vi "Test_Run All Tests.vi"(8 "error in":errorcluster, 9 "Modules":T7, 10 "Part Number":T9, 11 "Test Selection":T8) -> (0 "error out":errorcluster)   [LabVIEW 2025]
uses:
  Classes/Solenoid/Solenoid Selector.ctl
  Controls/Test list.ctl
  Controls/tests tab control.ctl
  Controls/Graphs/XY Graph_Transparent.ctl
  Controls/Test Results/Test Pass Fail.ctl
  Controls/Test Results/Results Table.ctl
  Controls/Numeric Voltage.ctl
  Controls/Numeric Current.ctl
  Classes/Solenoid/Solenoid.lvclass
  Classes/EVI 79/EVI 79.lvclass
  C:/Users/grove/Desktop/LabVIEW/Git/atp-station/Classes/Solenoid/Solenoid.lvclass
  Test_Calculate Wear-in.vi
  Test_Calculate Drop-out.vi
  Test_Calculate CRT.vi
  Test_Calculate Pull-in.vi
  Test_Calculate Hold-in.vi
  Test_Calculate ORT.vi
  Libraries/Power Supply/Power Supply.lvlib
  Libraries/USB IO/USB IO.lvlib
panel:
  out "Voltage Chart":dbl(graph)
  out "Current":T1 format="%5.3f A"
  out "Voltage":T2 format="%5.3f V"
  out "result 3":bool
  out "result 2":bool
  out "result":bool
  in  "Table Control":T3=[["Wear-in", "N/A", "N/A", "", "", "", "", ""], ["Drop-out", "N/A", "N/A", "", "", "", "", ""], ["Closing Response Time", "N/A", "N/A", "", "", "", "", ""], ["Pull-in", "N/A", "N/A", "", "", "", "", ""], ["Hold-in", "N/A", "N/A", "", "", "", "", ""], ["Opening Response Time", "N/A", "N/A", "", "", "", "", ""]]
  out "Errors":errorcluster
  in  "Tab Control":T4
  out "Power Supply Output":bool
  out "Cycles":dbl format="%3.0f of"
  out "Total Cycles":dbl format="%3.0f"
  out "Unit On?":bool
  in  "Abort":bool
  out "Drop-out Voltage":T2 format="%5.3f V"
  out "Drop-out Current":T1 format="%5.3f A"
  out "CRT Graph":T5
  out "Closing Response Time":dbl format="%5.3f ms"
  out "Pass? 2":T6 caption="Test Result"
  out "Pull-in Voltage":T2 format="%5.3f V"
  out "Pull-in Current":T1 format="%5.3f A"
  in  "Abort 2":bool
  out "XY Graph":T5
  out "Pass?":T6 caption="Test Result"
  out "Opening Response Time":dbl format="%5.3f ms"
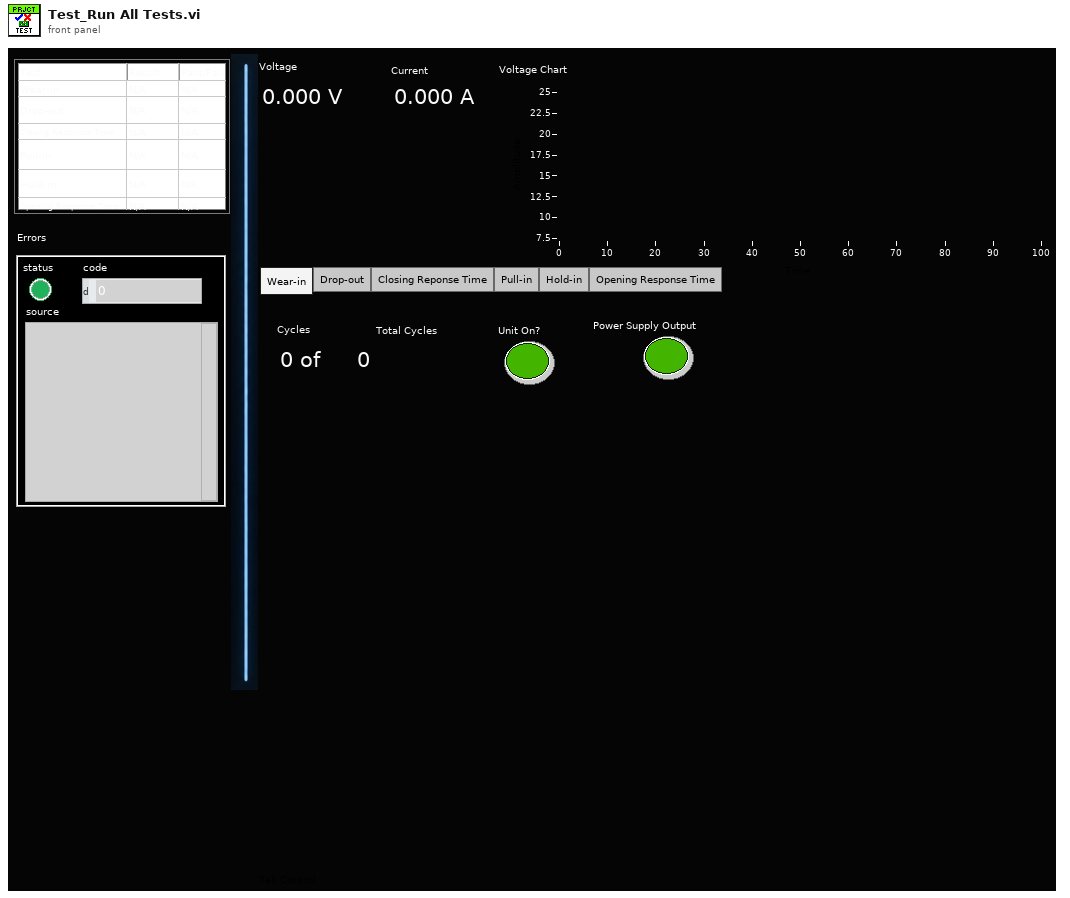
[diagram p1: front panel]
types:
  T1 = typedef "Numeric Current.ctl" = dbl
  T2 = typedef "Numeric Voltage.ctl" = dbl
  T3 = typedef "Results Table.ctl" = string[][]
  T4 = typedef "tests tab control.ctl" = enum32{"Wear-in", "Drop-out", "Closing Reponse Time", "Pull-in", "Hold-in", "Opening Response Time"}
  T5 = typedef "XY Graph_Transparent.ctl" = cluster{dbl[], dbl[]}[]
  T6 = typedef "Test Pass Fail.ctl" = bool
  T7 = cluster{"Module IDs":i32[], "Module Names":string[]}
  T8 = typedef "Test list.ctl" = cluster{"Wear-in":bool, "Drop-out":bool, "Closing Response Time":bool, "Pull-in":bool, "Hold-in":bool, "Opening Response Time":bool}
  T9 = typedef "Solenoid Selector.ctl" = enum16{"Generic Solenoid", "EVI-79"}
  T10 = cluster{"V":dbl, "I":dbl, "Cycles":dbl, "On_Time_ms":dbl, "Off_Time_ms":dbl}
  T11 = cluster{"V":dbl, "I":dbl, "V_reduced":dbl, "V_perturb":dbl, "Plunger_Threshold":dbl, "Plunger_Threshold 2":dbl}
  T12 = cluster{"V":dbl, "I":dbl, "V_increased":dbl, "V_perturb":dbl, "Plunger_Threshold":dbl, "V_MAX":dbl}
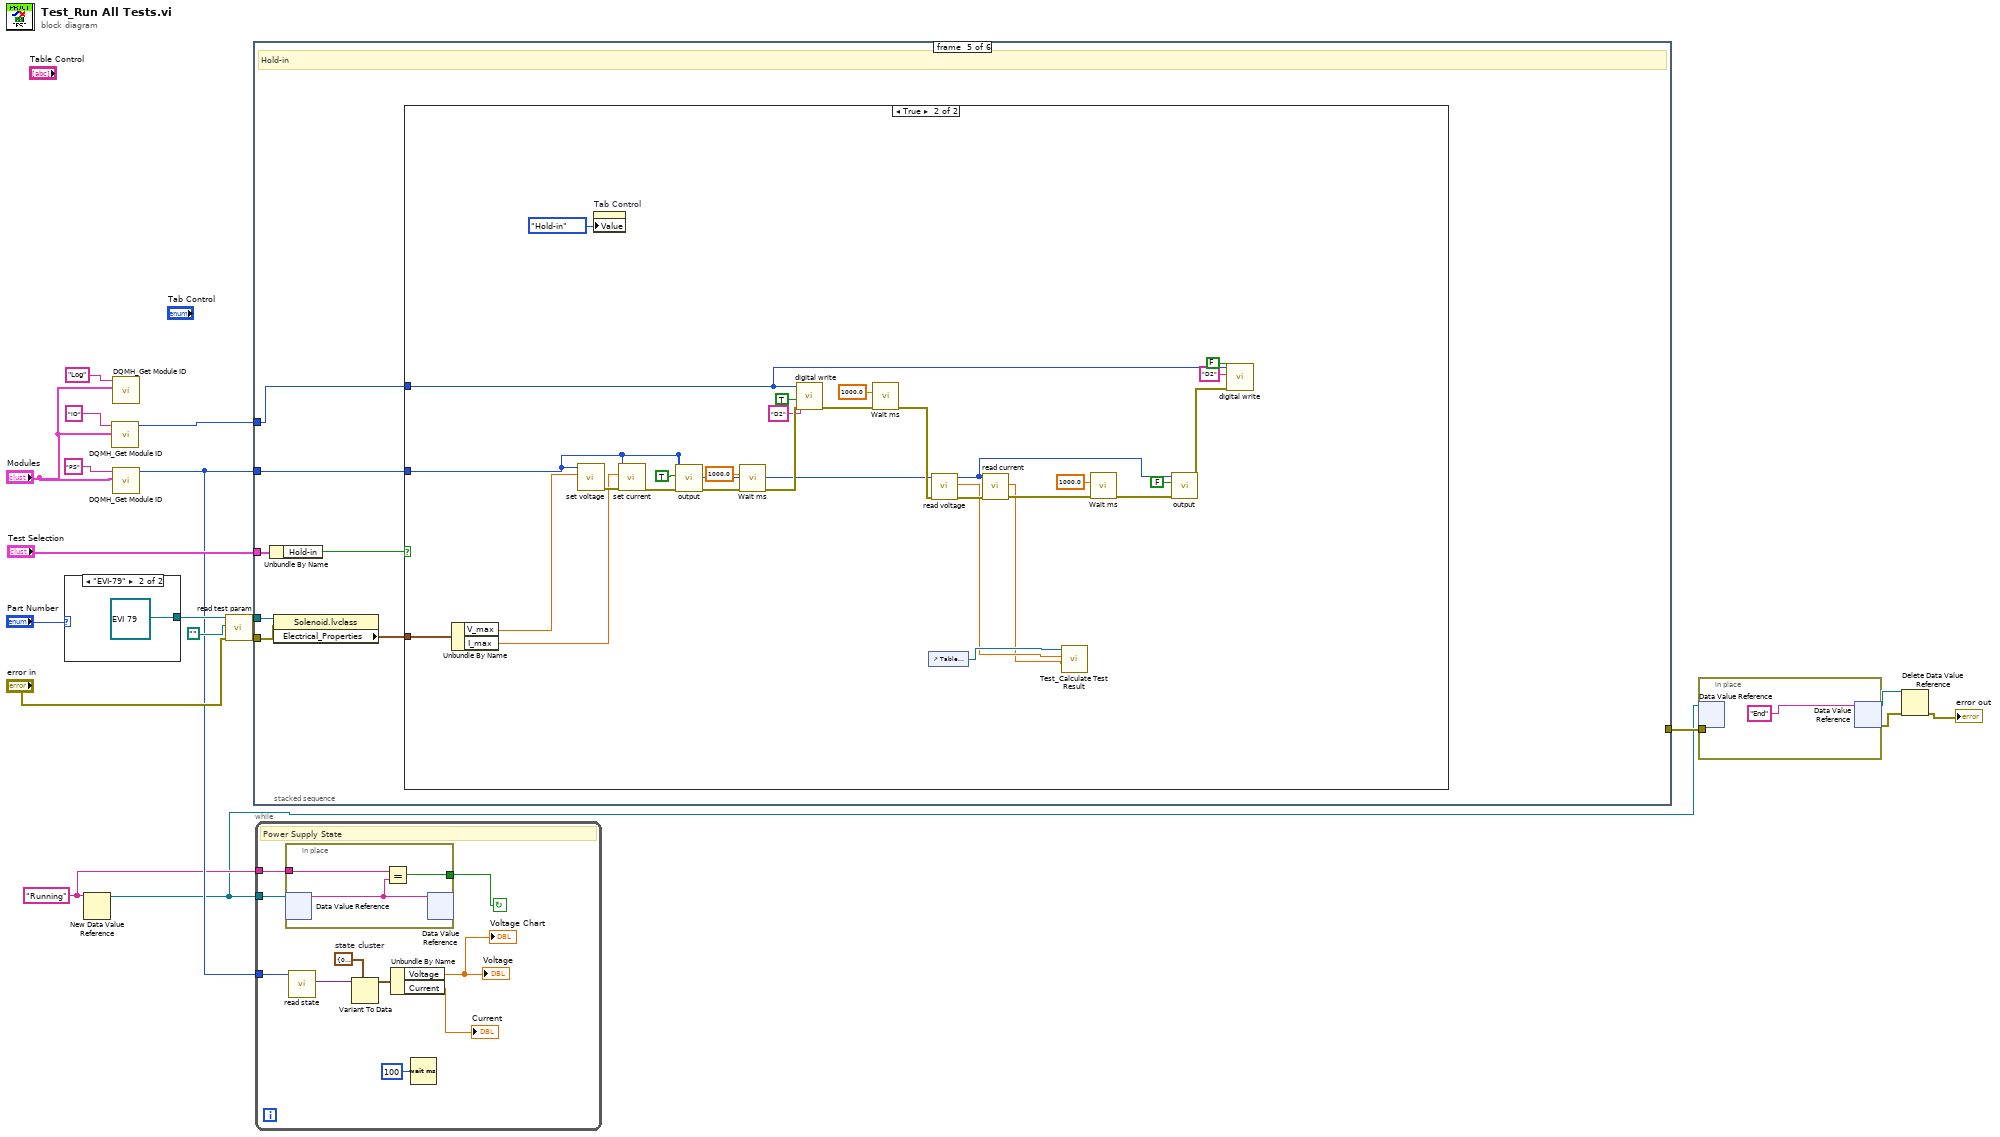
[diagram p0: block diagram]
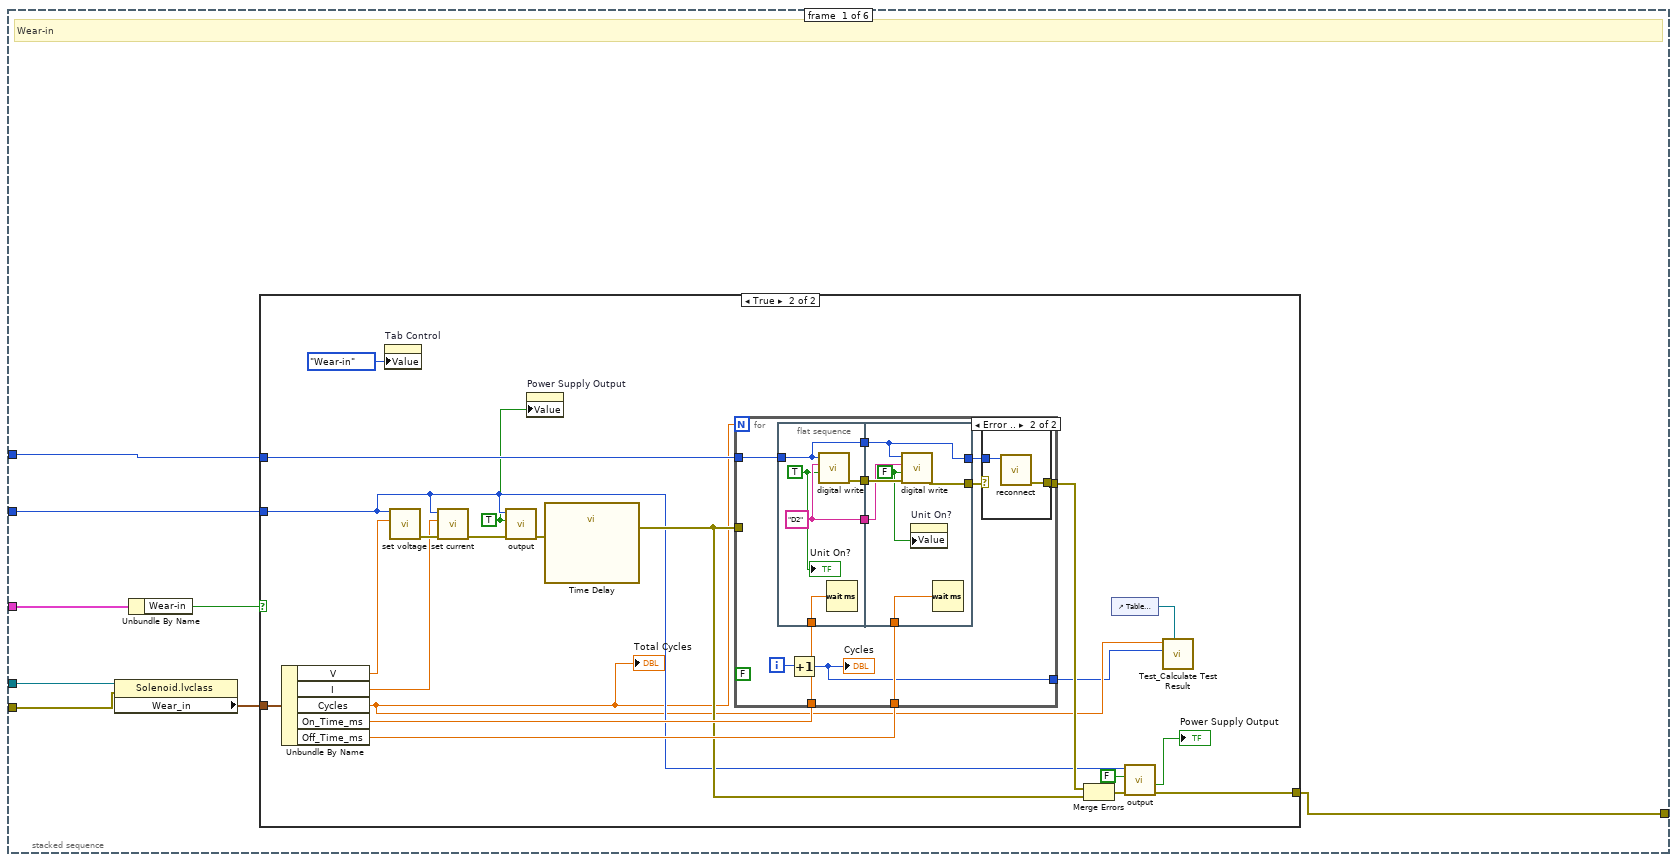
[diagram p2: hidden frame]
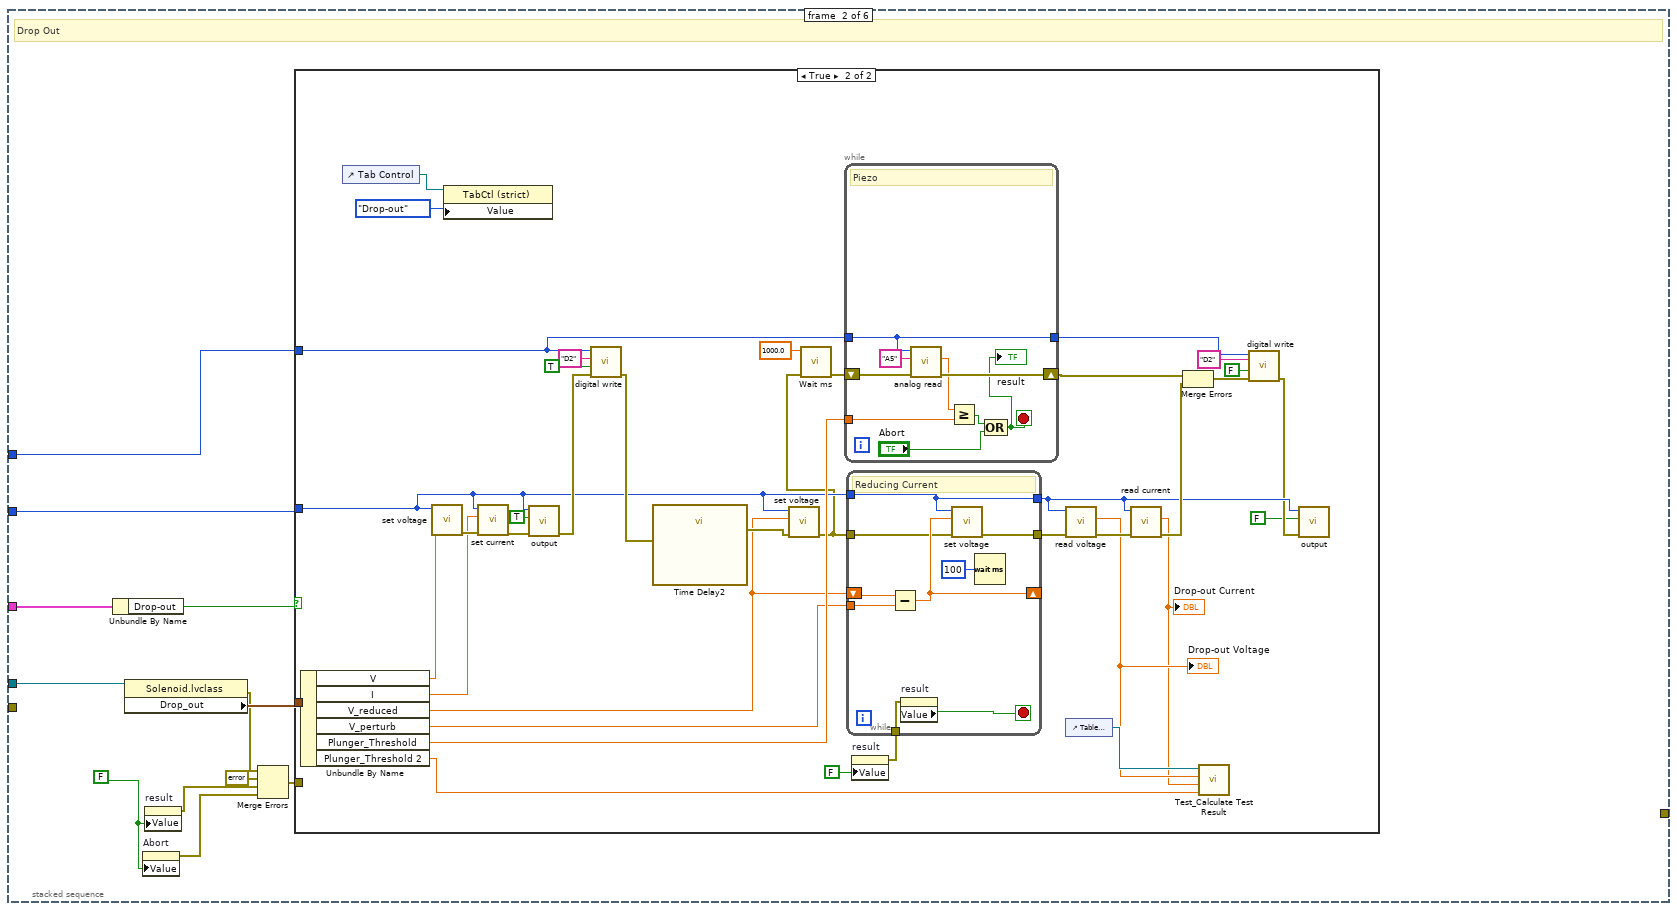
[diagram p5: hidden frame]
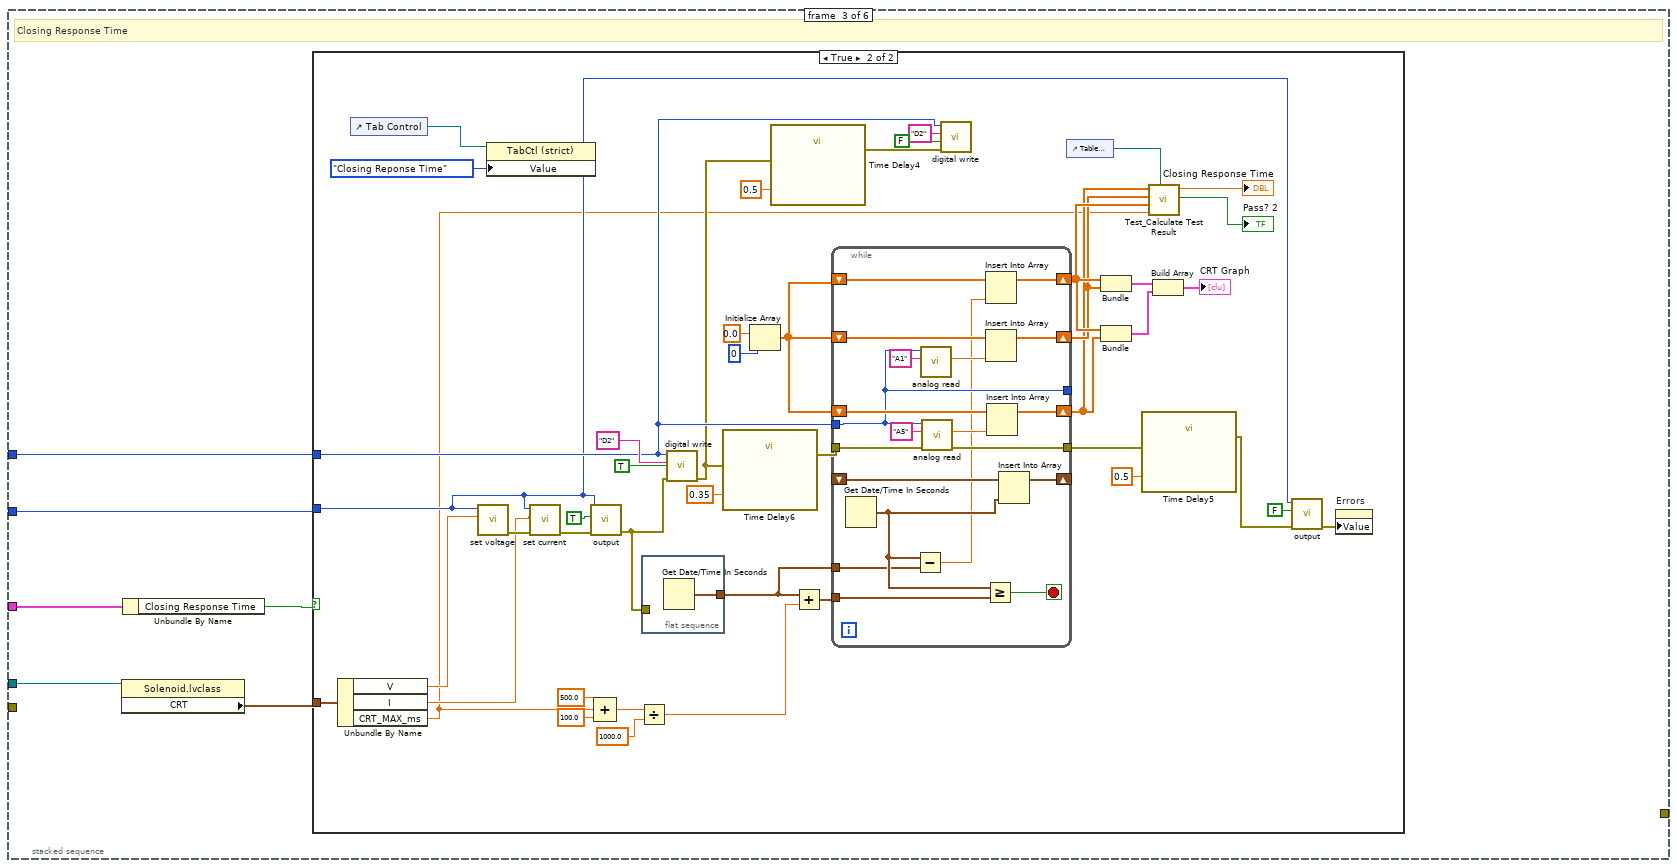
[diagram p7: hidden frame]
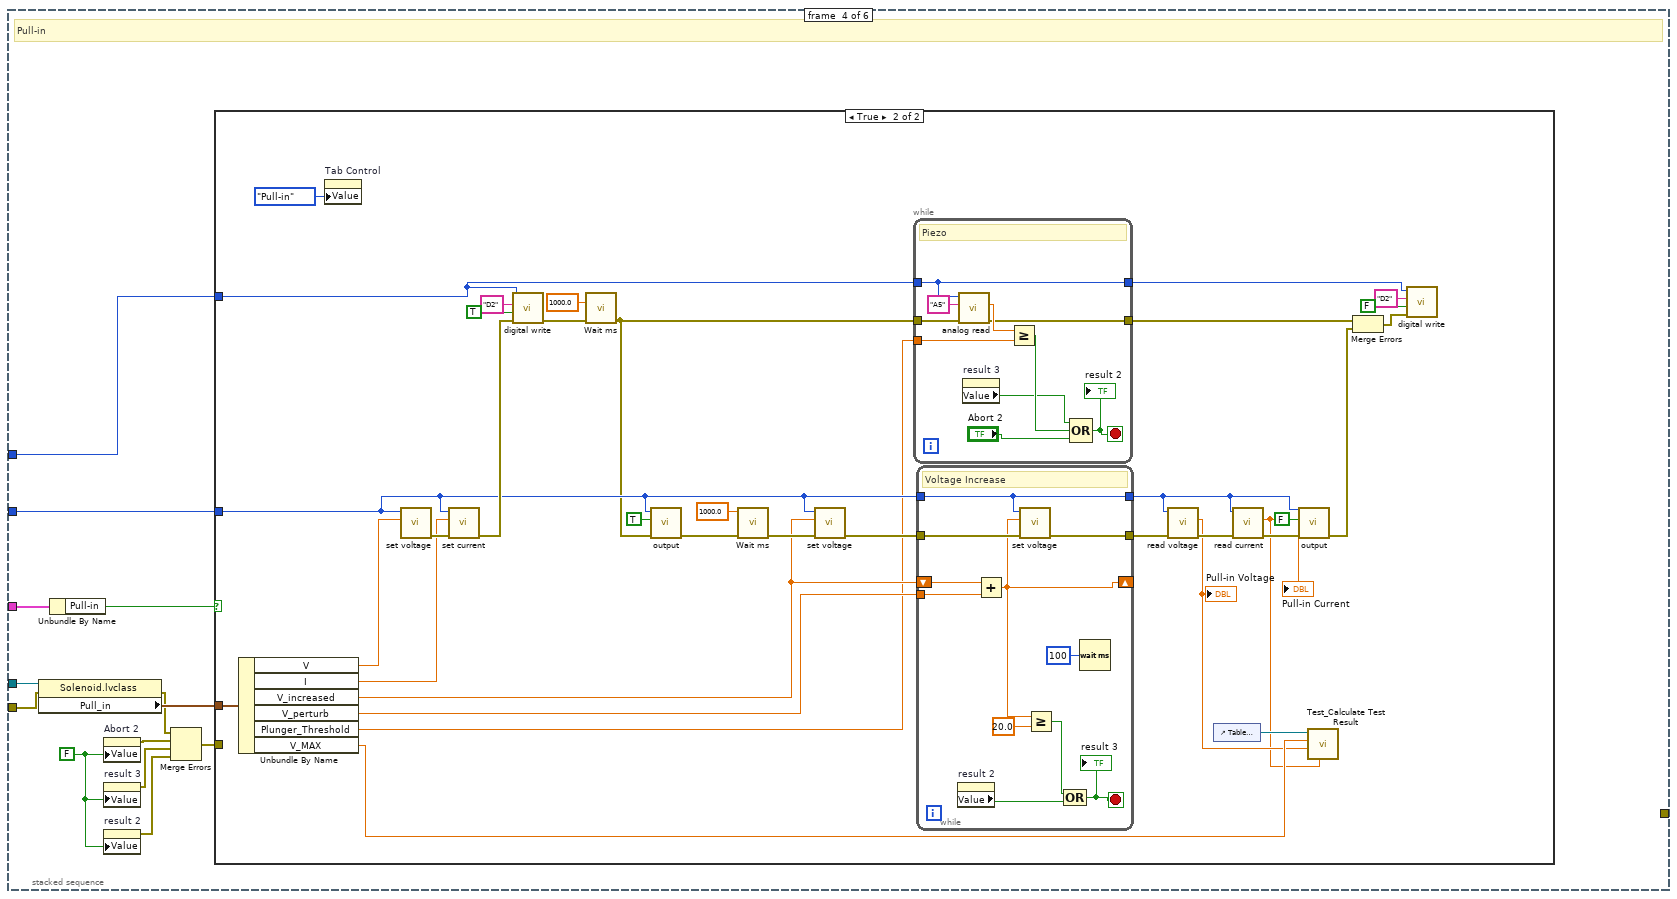
[diagram p9: hidden frame]
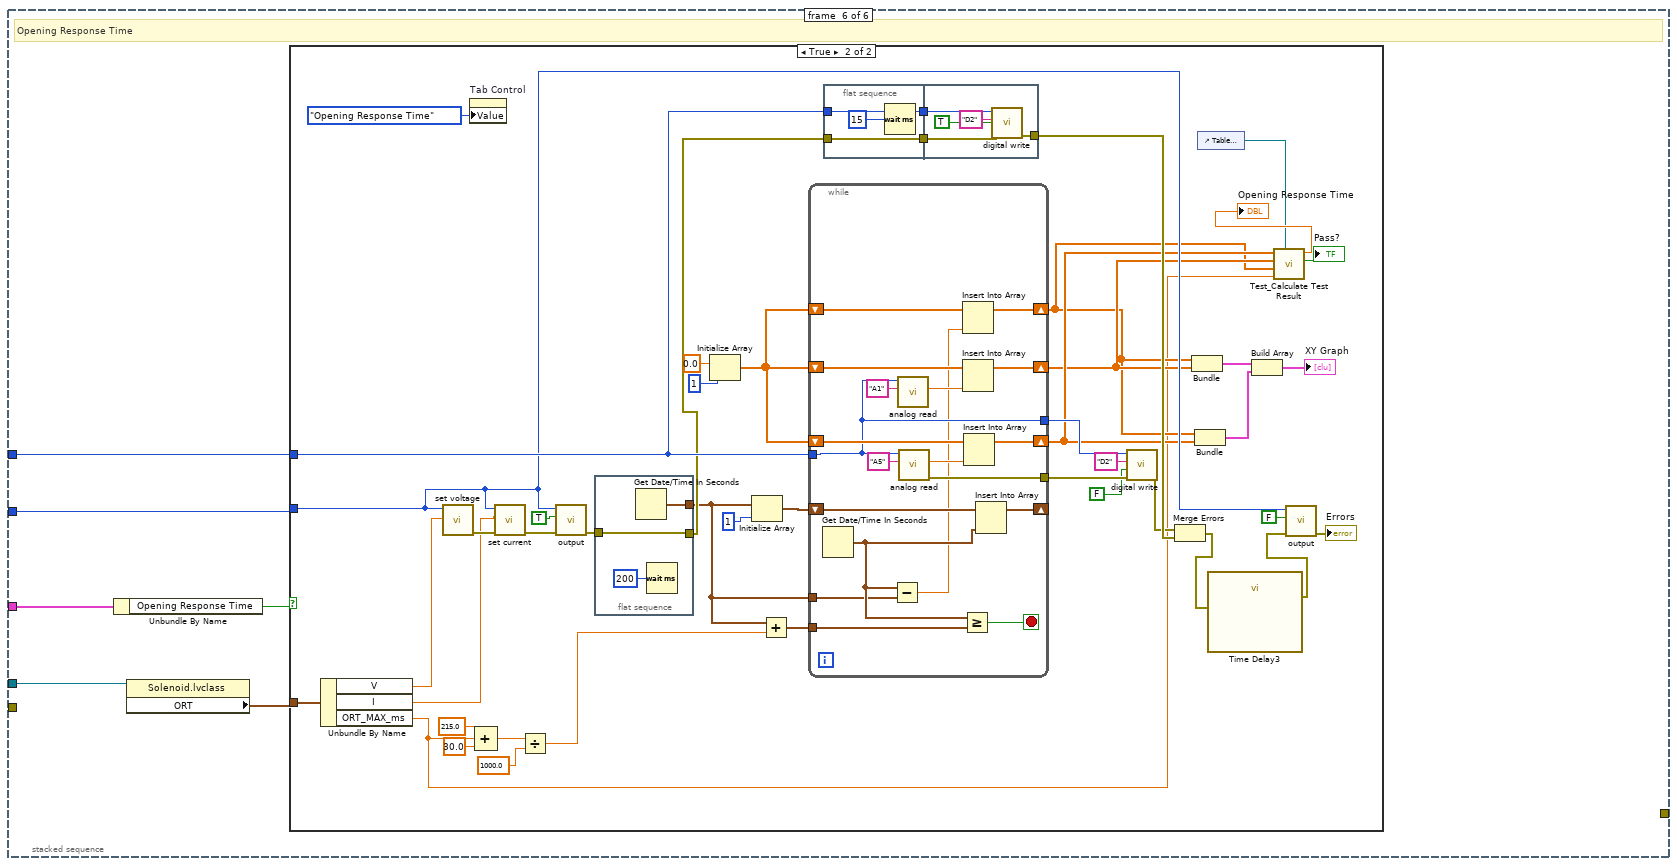
[diagram p12: hidden frame]
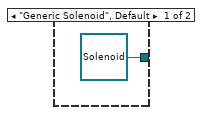
[diagram p14: hidden frame]
diagram:
  w6 = "Running"
  n1 = case shown="\"EVI-79\"" "Part Number" {
    tunnel: [refnum<class "Solenoid.lvclass"> refnum ("Solenoid.lvclass") refnum<class "EVI 79.lvclass"> refnum ("EVI 79.lvclass")] -> w18
    frame "Generic Solenoid", Default {
    }
    frame "EVI-79" {
    }
  }
  n2 = New Data Value Reference(data value=w6) -> (data value reference=w4:refnum<data-value>)  [unwired: 1 in, 1 out]
  n3 = call "DQMH_Get Module ID.vi"("Modules"="Modules", "Module Name"="IO") -> ("Module ID out"=w8:i32)  [unwired: 9 in]
  n4 = call "DQMH_Get Module ID.vi"("Modules"="Modules", "Module Name"="Log") -> ()  [unwired: 9 in, 1 out]
  n5 = call "DQMH_Get Module ID.vi"("Modules"="Modules", "Module Name"="PS") -> ("Module ID out"=w7:i32)  [unwired: 9 in]
  n6 = call-dynamic "read test param.vi"("error in (no error)"="error in", "File Path"=path "", "Solenoid in"=w18) -> ("error out"=w13:errorcluster, "Solenoid out"=w15:refnum<class "Solenoid.lvclass">)  [unwired: 7 in]
  n7 = stacked-sequence {
    tunnel: w15 -> [w27 w85 w147 w226 w290 w326]
    tunnel: "Test Selection" -> [w29 w87 w149 w228 w292 w325]
    tunnel: w13 -> [w26 _ _ w225 w289 _]
    tunnel: w7 -> [w24 w83 w145 w223 w287 w322]
    tunnel: w8 -> [w23 w82 w144 w222 w286 w321]
    tunnel: [w22 _ _ _ _ _] -> w5
    frame #0 {
      # "Wear-in"
      n8 = property class="Solenoid.lvclass"(reference=w27, error in=w26) -> ("Wear_in"=w25:T10)  [unwired: 2 out]
      n9 = Unbundle By Name(w29) -> ("Wear-in"=w28:bool)
      n10 = case shown="True" w28 {
        tunnel: w25 -> [_ w50]
        tunnel: w24 -> [_ w39]
        tunnel: w23 -> [_ w46]
        tunnel: [_ w40] -> w22
        frame False {
        }
        frame True {
          w37 = TRUE ("Output On/Off")
          n11 = Unbundle By Name(w50) -> ("V"=w32:dbl, "I"=w31:dbl, "Cycles"=w35:dbl, "On_Time_ms"=w48:dbl, "Off_Time_ms"=w47:dbl)
          "Total Cycles" <- w35
          n12 = property on="Tab Control" class="TabCtl (strict)"("Value"=tests_tab_control."Wear-in" ("Tab Control")) -> ()  [unwired: 2 in, 2 out]
          n13 = call "set voltage.vi"("Output Voltage"=w32, "Module ID"=w39) -> ("error out"=w49:errorcluster)  [unwired: 8 in, 1 out]
          n14 = call "set current.vi"("error in"=w49, "Output Current"=w31, "Module ID"=w39) -> ("error out"=w45:errorcluster)  [unwired: 7 in, 1 out]
          n15 = call "output.vi"("error in"=w45, "Output On/Off"=w37, "Module ID"=w39) -> ("error out"=w44:errorcluster)  [unwired: 7 in, 1 out]
          n16 = property on="Power Supply Output" class="Bool (strict)"("Value"=w37) -> ()  [unwired: 2 in, 2 out]
          n17 = call "Time Delay"("error in (no error)"=w44) -> ("error out"=w42:errorcluster)  [unwired: 10 in]
          n18 = for {
            N: w35 -> [_]
            tunnel: w48 -> [w61]
            tunnel: w47 -> [w60]
            tunnel: w46 -> [w59]
            tunnel: w42 -> [_]
            tunnel: [w53] -> w43
            tunnel: [w51] -> w34
            i -> [w55]
            (unwired) FALSE ("Power Supply Output")
            n19 = flat-sequence {
              tunnel: w61 -> [w69]
              tunnel: w59 -> [w67]
              tunnel: [w68] -> w58
              tunnel: [w67] -> w57
              tunnel: [w66] -> w56
              tunnel: w60 -> [w73]
              tunnel: w58 -> [w75]
              tunnel: w57 -> [w70]
              tunnel: w56 -> [w74]
              tunnel: [w72] -> w54
              tunnel: [w70] -> w52
              frame #0 {
                w65 = TRUE ("On/Off")
                w66 = "D2" ("Line")
                n20 = call "digital write.vi"("On/Off"=w65, "Line"=w66, "Module ID"=w67) -> ("error out"=w68:errorcluster)  [unwired: 7 in, 1 out]
                n21 = Wait (ms)(milliseconds to wait=w69) -> ()  [unwired: 1 out]
                "Unit On?" <- w65
              }
              frame #1 {
                w71 = FALSE ("On/Off")
                n22 = call "digital write.vi"("error in"=w75, "On/Off"=w71, "Line"=w74, "Module ID"=w70) -> ("error out"=w72:errorcluster)  [unwired: 6 in, 1 out]
                n23 = property on="Unit On?" class="Bool (strict)"("Value"=w71) -> ()  [unwired: 2 in, 2 out]
                n24 = Wait (ms)(milliseconds to wait=w73) -> ()  [unwired: 1 out]
              }
            }
            n25 = Increment(x=w55) -> (x+1=w51:i32)
            "Cycles" <- w51
            n26 = case shown="Error .." w54 {
              selector: w54 -> [w62 _]
              tunnel: [w62 w64] -> w53
              tunnel: w52 -> [_ w63]
              frame No Error {
              }
              frame Error {
                n27 = call "reconnect.vi"("Module ID"=w63) -> ("error out"=w64:errorcluster)  [unwired: 9 in, 1 out]
              }
            }
          }
          n28 = Merge Errors(w43, w42) -> (w41:errorcluster)
          n29 = control-ref of="Table Control"() -> (w33:refnum<vi>)
          n30 = call "output.vi"("error in"=w41, "Output On/Off"=FALSE, "Module ID"=w39) -> ("error out"=w40:errorcluster, "timed out?"=→"Power Supply Output":bool)  [unwired: 7 in]
          n31 = call-poly "Test_Calculate Test Result.vi"("Table Ref"=w33, "Cycles"=w34, "Total Cycles"=w35) -> ()  [unwired: 7 in, 2 out]
        }
      }
    }
    frame #1 {
      w81 = FALSE
      # "Drop Out"
      n32 = Unbundle By Name(w87) -> ("Drop-out"=w86:bool)
      n33 = property class="Solenoid.lvclass"(reference=w85) -> (error out=w80:errorcluster, "Drop_out"=w84:T11)  [unwired: 1 in, 1 out]
      n34 = property on="Abort" class="Bool (strict)"("Value"=w81) -> (error out=w78:errorcluster)  [unwired: 2 in, 1 out]
      n35 = property on="result" class="Bool (strict)"("Value"=w81) -> (error out=w79:errorcluster)  [unwired: 2 in, 1 out]
      n36 = Merge Errors(w80, errorcluster {"status"=FALSE, "code"=0, "source"=""} ("error in"), w79, w78) -> (w77:errorcluster)
      n37 = case shown="True" w86 {
        tunnel: w84 -> [_ w125]
        tunnel: w83 -> [_ w112]
        tunnel: w82 -> [_ w116]
        tunnel: w77 -> [_ _]
        frame False {
        }
        frame True {
          n38 = Unbundle By Name(w125) -> ("V"=w91:dbl, "I"=w90:dbl, "V_reduced"=w114:dbl, "V_perturb"=w113:dbl, "Plunger_Threshold"=w115:dbl, "Plunger_Threshold 2"=w97:dbl)
          n39 = control-ref of="Tab Control"() -> (w89:refnum<vi>)
          n40 = call "set voltage.vi"("Output Voltage"=w91, "Module ID"=w112) -> ("error out"=w124:errorcluster)  [unwired: 8 in, 1 out]
          n41 = property on="Property Node" class="TabCtl (strict)"(reference=w89, "Value"=tests_tab_control."Drop-out" ("Tab Control")) -> ()  [unwired: 1 in, 2 out]
          n42 = call "set current.vi"("error in"=w124, "Output Current"=w90, "Module ID"=w112) -> ("error out"=w123:errorcluster)  [unwired: 7 in, 1 out]
          n43 = call "output.vi"("error in"=w123, "Output On/Off"=TRUE, "Module ID"=w112) -> ("error out"=w121:errorcluster)  [unwired: 7 in, 1 out]
          n44 = call "digital write.vi"("error in"=w121, "On/Off"=TRUE, "Line"="D2", "Module ID"=w116) -> ("error out"=w117:errorcluster)  [unwired: 6 in, 1 out]
          n45 = call "Time Delay2"("error in (no error)"=w117) -> ("error out"=w118:errorcluster)  [unwired: 10 in]
          n46 = call "set voltage.vi"("error in"=w118, "Output Voltage"=w114, "Module ID"=w112) -> ("error out"=w95:errorcluster)  [unwired: 7 in, 1 out]
          n47 = call "Wait ms.vi"("error in (no error)"=w95, "Delay Time (ms)"=1000.0) -> ("error out"=w96:errorcluster)  [unwired: 9 in]
          n48 = while {
            tunnel: w116 -> [w139]
            shift-right: [w142] -> w109
            shift-left: w96 -> [w136]
            tunnel: w115 -> [w140]
            tunnel: [w139] -> w107
            stop <- w137 stop-if-true
            # "Piezo"
            n49 = call "analog read.vi"("error in"=w136, "Line"="A5", "Module ID"=w139) -> ("error out"=w142:errorcluster, "Voltage"=w141:T2)  [unwired: 6 in, 1 out]
            n50 = Greater Or Equal?(x=w141, y=w140) -> (x >= y?=w135:bool)
            n51 = Compound Arithmetic op=OR(w135, "Abort") -> (w137:bool)
            "result" <- w137
          }
          n52 = property on="result" class="Bool (strict)"("Value"=FALSE) -> (error out=w93:errorcluster)  [unwired: 2 in, 1 out]
          n53 = while {
            shift-right: [w129] -> _
            shift-left: w114 -> [w134]
            tunnel: w113 -> [w133]
            tunnel: w95 -> [w128]
            tunnel: w112 -> [w130]
            tunnel: [w132] -> w111
            tunnel: [w130] -> w104
            tunnel: w93 -> [w127]
            stop <- w126 stop-if-true
            # "Reducing Current"
            n54 = Subtract(x=w134, y=w133) -> (x-y=w129:dbl)
            n55 = property on="result" class="Bool (strict)"(error in=w127) -> ("Value"=w126:bool)  [unwired: 1 in, 2 out]
            n56 = call "set voltage.vi"("error in"=w128, "Output Voltage"=w129, "Module ID"=w130) -> ("error out"=w132:errorcluster)  [unwired: 7 in, 1 out]
            n57 = Wait (ms)(milliseconds to wait=u32 100) -> ()  [unwired: 1 out]
          }
          n58 = call "read voltage.vi"("error in"=w111, "Module ID"=w104) -> ("error out"=w110:errorcluster, "Volts"=w99:T2)  [unwired: 7 in, 1 out]
          "Drop-out Voltage" <- w99
          n59 = control-ref of="Table Control"() -> (w100:refnum<vi>)
          n60 = call "read current.vi"("error in"=w110, "Module ID"=w104) -> ("error out"=w108:errorcluster, "Amps"=w98:T1)  [unwired: 7 in, 1 out]
          "Drop-out Current" <- w98
          n61 = Merge Errors(w109, w108) -> (w103:errorcluster)
          n62 = call-poly "Test_Calculate Test Result.vi"("V_MIN"=w97, "Amps"=w98, "Volts"=w99, "Table in"=w100) -> ()  [unwired: 8 in]
          n63 = call "digital write.vi"("error in"=w103, "On/Off"=FALSE, "Line"="D2", "Module ID"=w107) -> ("error out"=w102:errorcluster)  [unwired: 6 in, 1 out]
          n64 = call "output.vi"("error in"=w102, "Output On/Off"=FALSE, "Module ID"=w104) -> ()  [unwired: 7 in, 2 out]
        }
      }
    }
    frame #2 {
      # "Closing Response Time"
      n65 = property class="Solenoid.lvclass"(reference=w147) -> ("CRT"=w146:cluster{"V":dbl, "I":dbl, "CRT_MAX_ms":dbl})  [unwired: 1 in, 2 out]
      n66 = Unbundle By Name(w149) -> ("Closing Response Time"=w148:bool)
      n67 = case shown="True" w148 {
        tunnel: w146 -> [_ w194]
        tunnel: w145 -> [_ w166]
        tunnel: w144 -> [_ w171]
        frame False {
        }
        frame True {
          n68 = Unbundle By Name(w194) -> ("V"=w189:dbl, "I"=w190:dbl, "CRT_MAX_ms"=w156:dbl)
          n69 = control-ref of="Tab Control"() -> (w151:refnum<vi>)
          n70 = call "set voltage.vi"("Output Voltage"=w189, "Module ID"=w166) -> ("error out"=w193:errorcluster)  [unwired: 8 in, 1 out]
          n71 = property on="Property Node" class="TabCtl (strict)"(reference=w151, "Value"=tests_tab_control."Closing Reponse Time" ("Tab Control")) -> ()  [unwired: 1 in, 2 out]
          n72 = call "set current.vi"("error in"=w193, "Output Current"=w190, "Module ID"=w166) -> ("error out"=w191:errorcluster)  [unwired: 7 in, 1 out]
          n73 = call "output.vi"("error in"=w191, "Output On/Off"=TRUE, "Module ID"=w166) -> ("error out"=w186:errorcluster)  [unwired: 7 in, 1 out]
          n74 = Compound Arithmetic op=ADD(500.0 ("value"), w156, 100.0 ("value")) -> (w183:dbl)
          n75 = Divide(x=w183, y=1000.0) -> (x/y=w179:dbl)
          n76 = flat-sequence {
            tunnel: w186 -> [_]
            tunnel: [w195] -> w180
            frame #0 {
              n77 = Get Date/Time In Seconds() -> (seconds since 1Jan1904=w195:timestamp)
            }
          }
          n78 = call "digital write.vi"("error in"=w186, "On/Off"=TRUE, "Line"="D2", "Module ID"=w171) -> ("error out"=w161:errorcluster)  [unwired: 6 in, 1 out]
          n79 = call "Time Delay6"("error in (no error)"=w161, "Delay Time (s)"=0.35) -> ("error out"=w160:errorcluster)  [unwired: 9 in]
          n80 = Initialize Array(0.0 ("element"), 0 ("dimension size")) -> (w176:dbl[])
          n81 = call "Time Delay4"("error in (no error)"=w161, "Delay Time (s)"=0.5) -> ("error out"=w174:errorcluster)  [unwired: 9 in]
          n82 = Add(x=w180, y=w179) -> (x+y=w181:timestamp)
          n83 = while {
            shift-right: [w208] -> w158
            shift-left: w176 -> [w215]
            shift-right: [w213] -> w157
            shift-left: w176 -> [w212]
            tunnel: w171 -> [w206]
            tunnel: [w207] -> w170
            tunnel: [w206] -> _
            shift-right: [w204] -> _
            shift-left: _ -> [w205]
            tunnel: w181 -> [w201]
            shift-right: [w200] -> w159
            shift-left: w176 -> [w199]
            tunnel: w180 -> [w197]
            tunnel: w160 -> [w196]
            stop <- w203 stop-if-true
            n84 = Get Date/Time In Seconds() -> (seconds since 1Jan1904=w202:timestamp)
            n85 = Subtract(x=w202, y=w197) -> (x-y=w198:dbl)
            n86 = call "analog read.vi"("Line"="A1", "Module ID"=w206) -> ("Voltage"=w214:T2)  [unwired: 7 in, 2 out]
            n87 = call "analog read.vi"("error in"=w196, "Line"="A5", "Module ID"=w206) -> ("error out"=w207:errorcluster, "Voltage"=w211:T2)  [unwired: 6 in, 1 out]
            n88 = Greater Or Equal?(x=w202, y=w201) -> (x >= y?=w203:bool)
            n89 = Insert Into Array(array=w199, new element=w198) -> (w200:dbl[])  [unwired: 1 in]
            n90 = Insert Into Array(array=w215, new element=w214) -> (w208:dbl[])  [unwired: 1 in]
            n91 = Insert Into Array(array=w212, new element=w211) -> (w213:dbl[])  [unwired: 1 in]
            n92 = Insert Into Array(array=w205, new element=w202) -> (w204:timestamp[])  [unwired: 1 in]
          }
          n93 = call "digital write.vi"("error in"=w174, "On/Off"=FALSE, "Line"="D2", "Module ID"=w171) -> ()  [unwired: 6 in, 2 out]
          n94 = control-ref of="Table Control"() -> (w152:refnum<vi>)
          n95 = Bundle(w159, w158) -> (w164:cluster{dbl[], dbl[]})  [unwired: 1 in]
          n96 = Bundle(w159, w157) -> (w163:cluster{dbl[], dbl[]})  [unwired: 1 in]
          n97 = call "Time Delay5"("error in (no error)"=w170, "Delay Time (s)"=0.5) -> ("error out"=w168:errorcluster)  [unwired: 9 in]
          n98 = call-poly "Test_Calculate Test Result.vi"("Table Ref"=w152, "CRT_MAX"=w156, "Time Data"=w159, "Current Data"=w158, "Piezo Data"=w157) -> ("Pass?"=→"Pass? 2":bool, "CRT [ms]"=→"Closing Response Time":dbl)  [unwired: 5 in]
          n99 = Build Array(w164, w163) -> (→"CRT Graph":cluster{dbl[], dbl[]}[])
          n100 = call "output.vi"("error in"=w168, "Output On/Off"=FALSE, "Module ID"=w166) -> ("error out"=w165:errorcluster)  [unwired: 7 in, 1 out]
          n101 = property on="Errors" class="Clust (strict)"("Value"=w165) -> ()  [unwired: 2 in, 2 out]
        }
      }
    }
    frame #3 {
      w217 = FALSE
      # "Pull-in"
      n102 = property class="Solenoid.lvclass"(reference=w226, error in=w225) -> (error out=w221:errorcluster, "Pull_in"=w224:T12)  [unwired: 1 out]
      n103 = Unbundle By Name(w228) -> ("Pull-in"=w227:bool)
      n104 = property on="Abort 2" class="Bool (strict)"("Value"=w217) -> (error out=w220:errorcluster)  [unwired: 2 in, 1 out]
      n105 = property on="result 3" class="Bool (strict)"("Value"=w217) -> (error out=w219:errorcluster)  [unwired: 2 in, 1 out]
      n106 = property on="result 2" class="Bool (strict)"("Value"=w217) -> (error out=w218:errorcluster)  [unwired: 2 in, 1 out]
      n107 = Merge Errors(w221, w220, w219, w218) -> (w216:errorcluster)
      n108 = case shown="True" w227 {
        tunnel: w224 -> [_ w262]
        tunnel: w223 -> [_ w249]
        tunnel: w222 -> [_ w247]
        tunnel: w216 -> [_ _]
        frame False {
        }
        frame True {
          n109 = Unbundle By Name(w262) -> ("V"=w261:dbl, "I"=w230:dbl, "V_increased"=w252:dbl, "V_perturb"=w251:dbl, "Plunger_Threshold"=w246:dbl, "V_MAX"=w233:dbl)
          n110 = property on="Tab Control" class="TabCtl (strict)"("Value"=tests_tab_control."Pull-in" ("Tab Control")) -> ()  [unwired: 2 in, 2 out]
          n111 = call "set voltage.vi"("Output Voltage"=w261, "Module ID"=w249) -> ("error out"=w264:errorcluster)  [unwired: 8 in, 1 out]
          n112 = call "set current.vi"("error in"=w264, "Output Current"=w230, "Module ID"=w249) -> ("error out"=w258:errorcluster)  [unwired: 7 in, 1 out]
          n113 = call "digital write.vi"("error in"=w258, "On/Off"=TRUE, "Line"="D2", "Module ID"=w247) -> ("error out"=w257:errorcluster)  [unwired: 6 in, 1 out]
          n114 = call "Wait ms.vi"("error in (no error)"=w257, "Delay Time (ms)"=1000.0) -> ("error out"=w248:errorcluster)  [unwired: 9 in]
          n115 = call "output.vi"("error in"=w248, "Output On/Off"=TRUE, "Module ID"=w249) -> ("error out"=w255:errorcluster)  [unwired: 7 in, 1 out]
          n116 = call "Wait ms.vi"("error in (no error)"=w255, "Delay Time (ms)"=1000.0) -> ("error out"=w253:errorcluster)  [unwired: 9 in]
          n117 = call "set voltage.vi"("error in"=w253, "Output Voltage"=w252, "Module ID"=w249) -> ("error out"=w250:errorcluster)  [unwired: 7 in, 1 out]
          n118 = while {
            tunnel: w248 -> [w285]
            tunnel: w247 -> [w276]
            tunnel: w246 -> [w280]
            tunnel: [w277] -> w236
            tunnel: [w276] -> w235
            stop <- w283 stop-if-true
            # "Piezo"
            n119 = call "analog read.vi"("error in"=w285, "Line"="A5", "Module ID"=w276) -> ("error out"=w277:errorcluster, "Voltage"=w281:T2)  [unwired: 6 in, 1 out]
            n120 = property on="result 3" class="Bool (strict)"() -> ("Value"=w278:bool)  [unwired: 2 in, 2 out]
            n121 = Greater Or Equal?(x=w281, y=w280) -> (x >= y?=w279:bool)
            n122 = Compound Arithmetic op=OR(w278, w279, "Abort 2") -> (w283:bool)
            "result 2" <- w283
          }
          n123 = while {
            shift-right: [w265] -> _
            shift-left: w252 -> [w275]
            tunnel: w251 -> [w274]
            tunnel: w250 -> [w272]
            tunnel: w249 -> [w266]
            tunnel: [w267] -> w244
            tunnel: [w266] -> w242
            stop <- w270 stop-if-true
            # "Voltage Increase"
            n124 = property on="result 2" class="Bool (strict)"() -> ("Value"=w271:bool)  [unwired: 2 in, 2 out]
            n125 = Add(x=w275, y=w274) -> (x+y=w265:dbl)
            n126 = call "set voltage.vi"("error in"=w272, "Output Voltage"=w265, "Module ID"=w266) -> ("error out"=w267:errorcluster)  [unwired: 7 in, 1 out]
            n127 = Greater Or Equal?(x=w265, y=20.0) -> (x >= y?=w268:bool)
            n128 = Compound Arithmetic op=OR(w268, w271) -> (w270:bool)
            "result 3" <- w270
            n129 = Wait (ms)(milliseconds to wait=u32 100) -> ()  [unwired: 1 out]
          }
          n130 = call "read voltage.vi"("error in"=w244, "Module ID"=w242) -> ("error out"=w245:errorcluster, "Volts"=w232:T2)  [unwired: 7 in, 1 out]
          "Pull-in Voltage" <- w232
          n131 = control-ref of="Table Control"() -> (w234:refnum<vi>)
          n132 = call "read current.vi"("error in"=w245, "Module ID"=w242) -> ("error out"=w243:errorcluster, "Amps"=w231:T1)  [unwired: 7 in, 1 out]
          "Pull-in Current" <- w231
          n133 = call "output.vi"("error in"=w243, "Output On/Off"=FALSE, "Module ID"=w242) -> ("error out"=w237:errorcluster)  [unwired: 7 in, 1 out]
          n134 = call-poly "Test_Calculate Test Result.vi"("Amps"=w231, "Volts"=w232, "V_MAX"=w233, "Table in"=w234) -> ()  [unwired: 8 in]
          n135 = Merge Errors(w236, w237) -> (w238:errorcluster)
          n136 = call "digital write.vi"("error in"=w238, "On/Off"=FALSE, "Line"="D2", "Module ID"=w235) -> ()  [unwired: 6 in, 2 out]
        }
      }
    }
    frame #4 {
      # "Hold-in"
      n137 = Unbundle By Name(w292) -> ("Hold-in"=w291:bool)
      n138 = property class="Solenoid.lvclass"(reference=w290, error in=w289) -> ("Electrical_Properties"=w288:cluster{"V_max":dbl, "I_max":dbl})  [unwired: 2 out]
      n139 = case shown="True" w291 {
        tunnel: w288 -> [_ w320]
        tunnel: w287 -> [_ w302]
        tunnel: w286 -> [_ w299]
        frame False {
        }
        frame True {
          n140 = Unbundle By Name(w320) -> ("V_max"=w318:dbl, "I_max"=w317:dbl)
          n141 = call "set voltage.vi"("Output Voltage"=w318, "Module ID"=w302) -> ("error out"=w319:errorcluster)  [unwired: 8 in, 1 out]
          n142 = property on="Tab Control" class="TabCtl (strict)"("Value"=tests_tab_control."Hold-in" ("Tab Control")) -> ()  [unwired: 2 in, 2 out]
          n143 = call "set current.vi"("error in"=w319, "Output Current"=w317, "Module ID"=w302) -> ("error out"=w315:errorcluster)  [unwired: 7 in, 1 out]
          n144 = call "output.vi"("error in"=w315, "Output On/Off"=TRUE, "Module ID"=w302) -> ("error out"=w313:errorcluster)  [unwired: 7 in, 1 out]
          n145 = call "Wait ms.vi"("error in (no error)"=w313, "Delay Time (ms)"=1000.0) -> ("error out"=w312:errorcluster)  [unwired: 9 in]
          n146 = call "digital write.vi"("error in"=w312, "On/Off"=TRUE, "Line"="D2", "Module ID"=w299) -> ("error out"=w309:errorcluster)  [unwired: 6 in, 1 out]
          n147 = call "Wait ms.vi"("error in (no error)"=w309, "Delay Time (ms)"=1000.0) -> ("error out"=w307:errorcluster)  [unwired: 9 in]
          n148 = control-ref of="Table Control"() -> (w296:refnum<vi>)
          n149 = call "read voltage.vi"("error in"=w307, "Module ID"=w302) -> ("error out"=w306:errorcluster, "Volts"=w295:T2)  [unwired: 7 in, 1 out]
          n150 = call "read current.vi"("error in"=w306, "Module ID"=w302) -> ("error out"=w305:errorcluster, "Amps"=w294:T1)  [unwired: 7 in, 1 out]
          n151 = call-poly "Test_Calculate Test Result.vi"("Amps"=w294, "Volts"=w295, "Table in"=w296) -> ()  [unwired: 9 in]
          n152 = call "Wait ms.vi"("error in (no error)"=w305, "Delay Time (ms)"=1000.0) -> ("error out"=w303:errorcluster)  [unwired: 9 in]
          n153 = call "output.vi"("error in"=w303, "Output On/Off"=FALSE, "Module ID"=w302) -> ("error out"=w300:errorcluster)  [unwired: 7 in, 1 out]
          n154 = call "digital write.vi"("error in"=w300, "On/Off"=FALSE, "Line"="D2", "Module ID"=w299) -> ()  [unwired: 6 in, 2 out]
        }
      }
    }
    frame #5 {
      # "Opening Response Time"
      n155 = Unbundle By Name(w325) -> ("Opening Response Time"=w324:bool)
      n156 = property class="Solenoid.lvclass"(reference=w326) -> ("ORT"=w323:cluster{"V":dbl, "I":dbl, "ORT_MAX_ms":dbl})  [unwired: 1 in, 2 out]
      n157 = case shown="True" w324 {
        tunnel: w323 -> [_ w371]
        tunnel: w322 -> [_ w348]
        tunnel: w321 -> [_ w352]
        frame False {
        }
        frame True {
          n158 = Unbundle By Name(w371) -> ("V"=w332:dbl, "I"=w331:dbl, "ORT_MAX_ms"=w333:dbl)
          n159 = call "set voltage.vi"("Output Voltage"=w332, "Module ID"=w348) -> ("error out"=w370:errorcluster)  [unwired: 8 in, 1 out]
          n160 = property on="Tab Control" class="TabCtl (strict)"("Value"=tests_tab_control."Opening Response Time" ("Tab Control")) -> ()  [unwired: 2 in, 2 out]
          n161 = Compound Arithmetic op=ADD(215.0 ("value"), w333, 30.0 ("value")) -> (w357:dbl)
          n162 = call "set current.vi"("error in"=w370, "Output Current"=w331, "Module ID"=w348) -> ("error out"=w368:errorcluster)  [unwired: 7 in, 1 out]
          n163 = Divide(x=w357, y=1000.0) -> (x/y=w354:dbl)
          n164 = call "output.vi"("error in"=w368, "Output On/Off"=TRUE, "Module ID"=w348) -> ("error out"=w355:errorcluster)  [unwired: 7 in, 1 out]
          n165 = flat-sequence {
            tunnel: [w382] -> w337
            tunnel: w355 -> [w381]
            tunnel: [w381] -> w350
            frame #0 {
              n166 = Get Date/Time In Seconds() -> (seconds since 1Jan1904=w382:timestamp)
              n167 = Wait (ms)(milliseconds to wait=u32 200) -> ()  [unwired: 1 out]
            }
          }
          n168 = Initialize Array(0.0 ("element"), 1 ("dimension size")) -> (w341:dbl[])
          n169 = Initialize Array(w337, 1 ("dimension size")) -> (w360:timestamp[])
          n170 = Add(x=w337, y=w354) -> (x+y=w353:timestamp)
          n171 = while {
            shift-right: [w394] -> w335
            shift-left: w341 -> [w401]
            shift-right: [w399] -> w336
            shift-left: w341 -> [w398]
            tunnel: w352 -> [w392]
            tunnel: [w393] -> w365
            tunnel: [w392] -> w364
            shift-right: [w390] -> _
            shift-left: w360 -> [w391]
            tunnel: w353 -> [w387]
            shift-right: [w386] -> w334
            shift-left: w341 -> [w385]
            tunnel: w337 -> [w383]
            stop <- w389 stop-if-true
            n172 = Get Date/Time In Seconds() -> (seconds since 1Jan1904=w388:timestamp)
            n173 = Subtract(x=w388, y=w383) -> (x-y=w384:dbl)
            n174 = call "analog read.vi"("Line"="A1", "Module ID"=w392) -> ("Voltage"=w400:T2)  [unwired: 7 in, 2 out]
            n175 = call "analog read.vi"("Line"="A5", "Module ID"=w392) -> ("error out"=w393:errorcluster, "Voltage"=w397:T2)  [unwired: 7 in, 1 out]
            n176 = Greater Or Equal?(x=w388, y=w387) -> (x >= y?=w389:bool)
            n177 = Insert Into Array(array=w385, new element=w384) -> (w386:dbl[])  [unwired: 1 in]
            n178 = Insert Into Array(array=w401, new element=w400) -> (w394:dbl[])  [unwired: 1 in]
            n179 = Insert Into Array(array=w398, new element=w397) -> (w399:dbl[])  [unwired: 1 in]
            n180 = Insert Into Array(array=w391, new element=w388) -> (w390:timestamp[])  [unwired: 1 in]
          }
          n181 = flat-sequence {
            tunnel: w352 -> [w374]
            tunnel: [w374] -> w351
            tunnel: w350 -> [w372]
            tunnel: [w372] -> w349
            tunnel: w351 -> [w377]
            tunnel: w349 -> [w376]
            tunnel: [w375] -> w347
            frame #0 {
              n182 = Wait (ms)(milliseconds to wait=u32 15) -> ()  [unwired: 1 out]
            }
            frame #1 {
              n183 = call "digital write.vi"("error in"=w376, "On/Off"=TRUE, "Line"="D2", "Module ID"=w377) -> ("error out"=w375:errorcluster)  [unwired: 6 in, 1 out]
            }
          }
          n184 = call "digital write.vi"("error in"=w365, "On/Off"=FALSE, "Line"="D2", "Module ID"=w364) -> ("error out"=w346:errorcluster)  [unwired: 6 in, 1 out]
          n185 = Merge Errors(w346, w347) -> (w343:errorcluster)
          n186 = Bundle(w334, w335) -> (w340:cluster{dbl[], dbl[]})  [unwired: 1 in]
          n187 = Bundle(w334, w336) -> (w339:cluster{dbl[], dbl[]})  [unwired: 1 in]
          n188 = control-ref of="Table Control"() -> (w328:refnum<vi>)
          n189 = call "Time Delay3"("error in (no error)"=w343) -> ("error out"=w342:errorcluster)  [unwired: 10 in]
          n190 = Build Array(w340, w339) -> (→"XY Graph":cluster{dbl[], dbl[]}[])
          n191 = call-poly "Test_Calculate Test Result.vi"("Table Ref"=w328, "ORT_MAX"=w333, "Time Data"=w334, "Current Data"=w335, "Piezo Data"=w336) -> ("Pass?"=→"Pass?":bool, "ORT [ms]"=→"Opening Response Time":dbl)  [unwired: 5 in]
          n192 = call "output.vi"("error in"=w342, "Output On/Off"=FALSE, "Module ID"=w348) -> ("error out"=→"Errors":errorcluster)  [unwired: 7 in, 1 out]
        }
      }
    }
  }
  n193 = while {
    tunnel: w7 -> [w411]
    tunnel: w4 -> [w405]
    tunnel: w6 -> [w404]
    stop <- w403 continue-if-true
    w409 = cluster{"Voltage":dbl, "Current":dbl} {"Voltage"=0.0, "Current"=0.0}  # state cluster
    # "Power Supply State"
    n194 = in-place {
      in-place-border: w404 -> [w413]
      in-place-border: [w412] -> w403
      n195 = in-place-dvr #1(w405) -> (w414:string)  [unwired: 1 out]
      n196 = Equal?(x=w413, y=w414) -> (x = y?=w412:bool)
      n197 = in-place-dvr #1(w414) -> ()  [unwired: 2 out]
    }
    n198 = call "read state.vi"("Module ID"=w411) -> ("Variant"=w410:variant)  [unwired: 8 in, 2 out]
    n199 = Variant To Data(type=w409, Variant=w410) -> (data=w408:cluster{"Voltage":dbl, "Current":dbl})  [unwired: 1 in, 1 out]
    n200 = Unbundle By Name(w408) -> ("Voltage"=→"Voltage" →"Voltage Chart":dbl, "Current"=→"Current":dbl)
    n201 = Wait (ms)(milliseconds to wait=u32 100) -> ()  [unwired: 1 out]
  }
  n202 = in-place {
    in-place-border: w5 -> [_]
    n203 = in-place-dvr #2(w4) -> ()  [unwired: 2 out]
    n204 = in-place-dvr #2("End") -> (w2:refnum<data-value>, w3:errorcluster)
  }
  n205 = Delete Data Value Reference(data value reference=w2, error in=w3) -> (error out=→"error out":errorcluster)  [unwired: 1 out]
